vi "Load_from_DB_subVi.vi"(8 "error in (no error)":errorcluster, 10 "Wybranie bazy danych - plik .UDL":path, 11 "Wybranie tabeli z bazy danych":string) -> (0 "error out":errorcluster, 3 "data":T1(array[cluster]))   [LabVIEW 2019]
doc: "This Vi provides data to be loaded from DB. The input is source - Data Base path, .UDL file, Table name - we need to know from which table we want to load from. This Vi don't parametrize other select options, so this load like \" Select * from /table_name/.\nThe last input is error in. The outputs are the data recieved and error out."
uses:
  <vilib>/addons/database/Connection.llb/DB Tools Open Connec (Path).vi
  <vilib>/addons/database/_DB Variant To Data/Database Variant To Data.xnode
  <vilib>/addons/database/NI_Database_API.lvlib
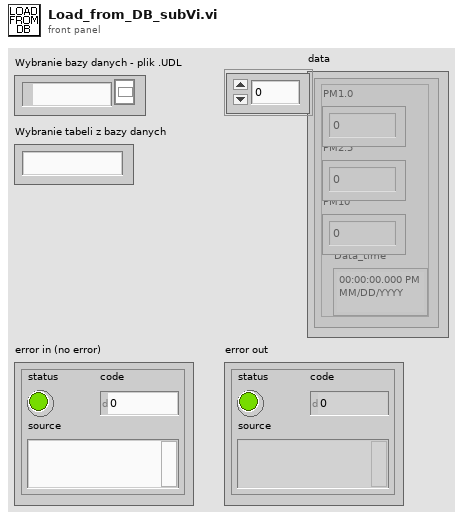
[diagram p1: front panel]
types:
  T1 = cluster{"PM1.0":i32, "PM2.5":i32, "PM10":i32, "Data_time":timestamp}[]
  T2 = typedef "NI_Database_API.lvlib/Conn ObjectReference.ctl" = refnum<k1>
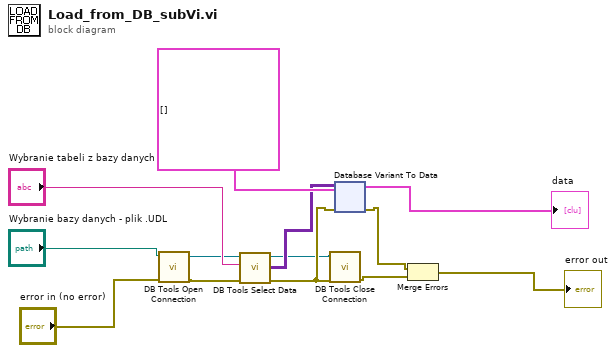
[diagram p0: block diagram]
diagram:
  n1 = call-poly <vilib>:"DB Tools Open Connection.vi"("error in (no error)"="error in (no error)", "connection information"="Wybranie bazy danych - plik .UDL") -> ("error out"=w2:errorcluster, "connection reference"=w3:T2)  [unwired: 6 in]
  n2 = call <vilib>:"DB Tools Select Data.vi"("error in (no error)"=w2, "table"="Wybranie tabeli z bazy danych", "connection reference"=w3) -> ("error out"=w9:errorcluster, "data"=w10:variant[][], "connection reference out"=w7:T2)  [unwired: 3 in]
  n3 = call <vilib>:"DB Tools Close Connection.vi"("error in (no error)"=w9, "connection reference"=w7) -> ("error out"=w4:errorcluster)  [unwired: 5 in]
  n4 = xnode "Database Variant To Data"("database variant"=w10, "error in (no error)"=w9, "type"=T1 []) -> ("data"=→"data":T1, "error out"=w8:errorcluster)
  n5 = Merge Errors(w8, w4) -> (→"error out":errorcluster)
